vi "AcceptDateSelection.vi"(8 "error in (no error)":errorcluster, 10 "Coords":T1, 11 "Calendar in":refnum<class "Calendar.lvclass">) -> (0 "error out":errorcluster, 1 "Accept?":bool, 2 "Day of Month":i32, 3 "Calendar (dup)":refnum<class "Calendar.lvclass">)   [LabVIEW 2015, in "Calendar.lvclass"]
uses:
  Calendar.lvclass
  <vilib>/Utility/miscctls.llb/LVPoint32TypeDef.ctl
  Calendar.lvclass/Calendar.ctl
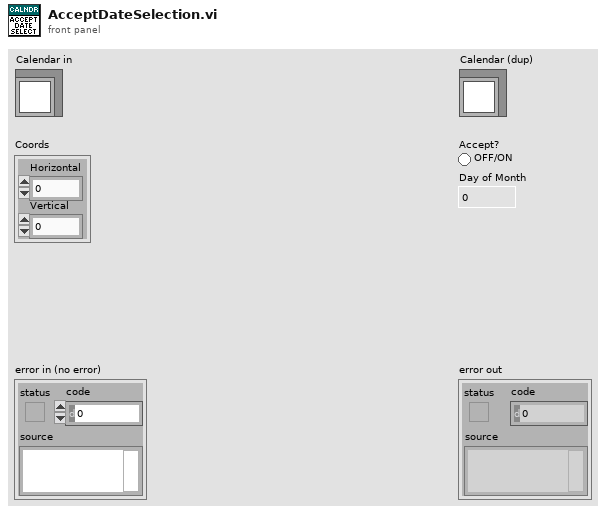
[diagram p1: front panel]
types:
  T1 = typedef "LVPoint32TypeDef.ctl" = cluster{"Horizontal":i32, "Vertical":i32}
  T2 = typedef "LVRowAndColumnTypeDef.ctl" = cluster{"Row":i32, "Column":i32}
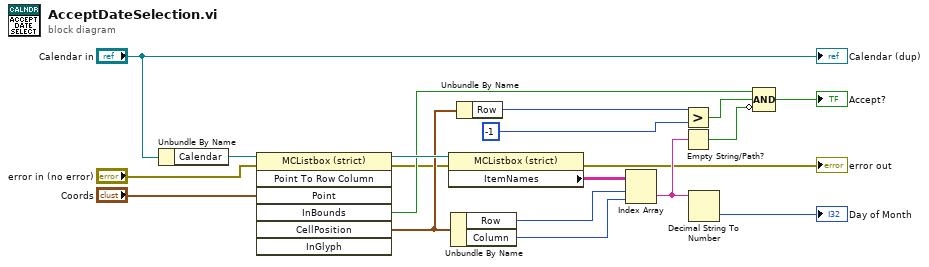
[diagram p0: block diagram]
diagram:
  n1 = Unbundle By Name("Calendar in") -> ("Calendar"=w18:refnum<vi>)
  n2 = invoke class="MCListbox (strict)" method="Point To Row Column"(reference=w18, error in="error in (no error)", "Point"="Coords") -> (reference out=w7:refnum<vi>, error out=w4:errorcluster, "InBounds"=w6:bool, "CellPosition"=w5:T2)  [unwired: 4 in, 3 out]
  n3 = property on="Property Node" class="MCListbox (strict)"(reference=w7, error in=w4) -> (error out=→"error out":errorcluster, "ItemNames"=w11:string[][])  [unwired: 1 out]
  n4 = Unbundle By Name(w5) -> ("Row"=w12:i32, "Column"=w13:i32)
  n5 = Unbundle By Name(w5) -> ("Row"=w15:i32)
  n6 = Index Array(array=w11, index (row)=w12, index (col)=w13) -> (element=w16:string)
  n7 = Greater?(x=w15, y=-1) -> (0:w9:bool)
  n8 = Empty String/Path?(string/path=w16) -> (empty?=w8:bool)
  n9 = Decimal String To Number(string=w16) -> (number=→"Day of Month":i32)  [unwired: 3 out]
  n10 = Compound Arithmetic op=AND(w6, w9, invert w8) -> (→"Accept?":bool)
  "Calendar (dup)" <- "Calendar in"
